vi "Register Panel Events.vi"(8 "error in (no error)":errorcluster, 10 "Event Refnum In":refnum<event-registration>, 11 "Panel Form Controller in":refnum<class "Panel Form Controller.lvclass">) -> (0 "error out":errorcluster, 2 "Event Refnum Out":refnum<event-registration>, 3 "Panel Form Controller out":refnum<class "Panel Form Controller.lvclass">)   [LabVIEW 2020, in "Panel Form Controller.lvlib" / "Panel Form Controller.lvclass"]
uses:
  Panel Form Controller.lvclass
  Panel Form Controller.lvclass/Panel Form Controller.ctl
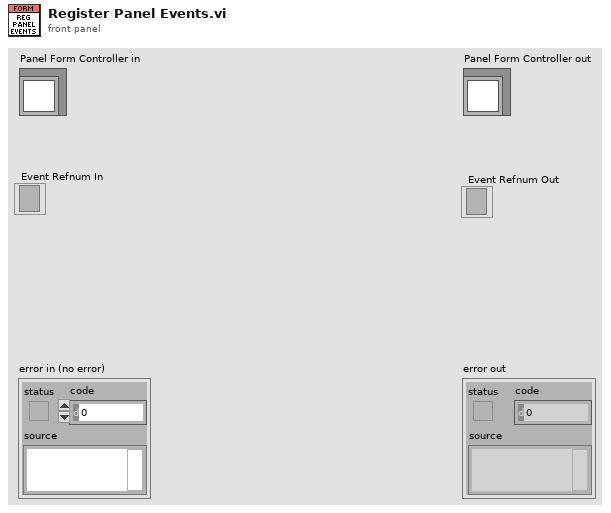
[diagram p1: front panel]
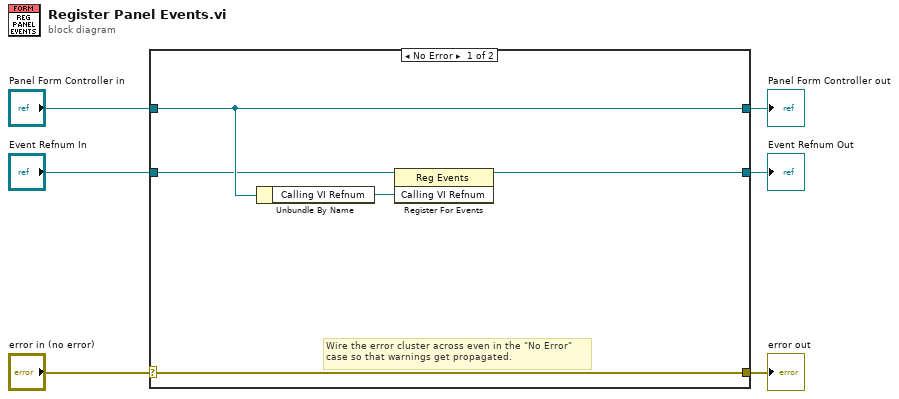
[diagram p0: block diagram]
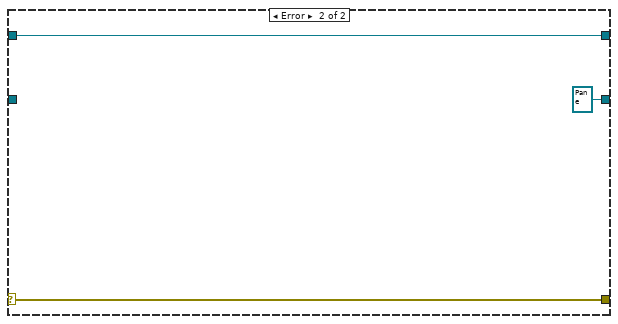
[diagram p2: hidden frame]
diagram:
  n1 = case shown="No Error" "error in (no error)" {
    selector: "error in (no error)" -> [w11 w14]
    tunnel: [w11 w14] -> w5
    tunnel: [w10 w13] -> w3
    tunnel: "Panel Form Controller in" -> [w10 w13]
    tunnel: [w9 refnum<event-registration> refnum ("Event Registration Refnum")] -> w2
    tunnel: "Event Refnum In" -> [w7 _]
    frame No Error {
      # "Wire the error cluster across even in the \"No Error\"\ncase so that warnings get propagated."
      n2 = Unbundle By Name(w10) -> ("Calling VI Refnum"=w8:refnum<vi>)
      n3 = register-events(reference=w7, w8) -> (reference out=w9:refnum<event-registration>)  [unwired: 1 in, 1 out]
    }
    frame Error {
    }
  }
  "error out" <- w5
  "Panel Form Controller out" <- w3
  "Event Refnum Out" <- w2
